vi "JKISM++ Global Log Event.vi"(8 "Error in":errorcluster caption="Error in (no error)") -> (0 "Error out":errorcluster, 3 "JKISM Global Log Event":refnum<user-event>)   [LabVIEW 2014, in "JKI State Machine++.lvlib"]
doc: "获取 JKISM 全局状态用户事件句柄\n\n<b>输入控件:</b>\n - <b>Error in</b>: 错误簇\n\n<b>输出控件:</b>\n - <b>JKISM Global Log Event</b>: JKISM 全局状态用户事件句柄\n - <b>Error out</b>: 错误簇"
uses:
  JKI State Machine++.lvlib
  _Support/Typedef/_JKISM Current State.ctl
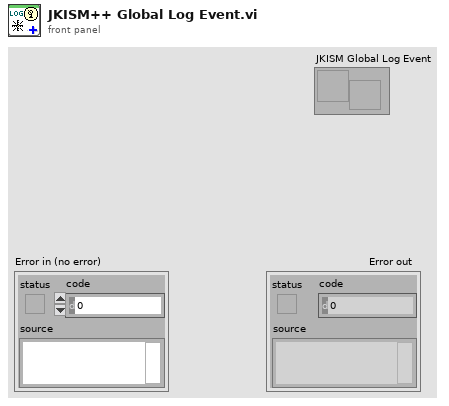
[diagram p1: front panel]
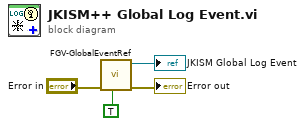
[diagram p0: block diagram]
diagram:
  n1 = call "FGV-GlobalEventRef.vi"("Create(F)"=TRUE, "error in (no error)"="Error in") -> ("error out"=→"Error out":errorcluster, "JKISM Global Log Event"=→"JKISM Global Log Event":refnum<user-event>)  [unwired: 8 in]
